vi "Adressen.vi"(8 "error in (no error)":errorcluster caption="Fehler (Eingang, kein Fehler)", 11 "Schneider Steuerung PNS Eingang":refnum<class "Schneider Steuerung PNS.lvclass">) -> (0 "error out":errorcluster caption="Fehler (Ausgang)", 2 "Adressen out":T1, 3 "Schneider Steuerung PNS Ausgang":refnum<class "Schneider Steuerung PNS.lvclass">)   [LabVIEW 2020, in "Schneider Steuerung PNS.lvclass"]
uses:
  Schneider Steuerung PNS.lvclass
  Adresse.ctl
  Steuerung PNS.lvclass
panel:
  in  "Adressen IP":i32[](array[numeric])=[4000, 4001, 4002, 4003, 4090]
  in  "Alarm":i32[](array[numeric])=[300, 200, 301, 201, 302, 202, 303, 203, 304, 204, 305, 205, 306, 206, 307, 207]
  in  "Heizkreiserkennung":i32[](array[numeric])=[520, 521, 522, 523, 524, 525, 526, 527]
  in  "Allgemein":i32[](array[numeric])=[504, 506, 503, 502, 501, 500, 870, 4976, 505, 4977, 4978, 4979, 4980, 5000, 5002]
  in  "Loop 8":i32[](array[numeric])=[407, 7, 207, 307, 457, 107]
  in  "Loop 7":i32[](array[numeric])=[406, 6, 206, 306, 456, 106]
  in  "Loop 6":i32[](array[numeric])=[405, 5, 205, 305, 455, 105]
  in  "Loop 5":i32[](array[numeric])=[404, 4, 204, 304, 454, 104]
  in  "Loop 4":i32[](array[numeric])=[403, 3, 203, 303, 453, 103]
  in  "Loop 3":i32[](array[numeric])=[402, 2, 202, 302, 452, 102]
  in  "Loop 2":i32[](array[numeric])=[401, 1, 201, 301, 451, 101]
  in  "Loop 1":i32[](array[numeric])=[400, 8, 200, 300, 450, 100]
  # "Istwert\n\nSollwert\n\nAlarm MIN\n\nAlarm MAX\n\nRegler sperren\n\nAnalog Ausgang"
  # "AWC ist\n\nAusgang Prop.\n\nAuswahl NW/M/BP\n\nAWC Netzwerk\n\nAWC Manuell\n\nAWC Bitparallel\n\nDruckluft störung\n\nGeräte Erkennung\n\nGeräte Type\n\nSeriennummer\n\nIB-Jahr\n\nSoftWare Version\n\nLP Kennung\n\nVentile Schalten\n\nVentilstellung Anzeige"
  # "Benennung Heizkreis 1\n\nBenennung Heizkreis 2\n\nBenennung Heizkreis 3\n\nBenennung Heizkreis 4\n\nBenennung Heizkreis 5\n\nBenennung Heizkreis 6\n\nBenennung Heizkreis 7\n\nBenennung Heizkreis 8"
  # "Alarm Filter max\n\nAlarm Filter min\n\nAlarm Ventilplatte max\n\nAlarm Ventilplatte min\n\nAlarm HL1 max\n\nAlarm HL1 min\n\nAlarm HL2 max\n\nAlarm HL2 min\n\nAlarm HL3 max\n\nAlarm HL3 min\n\nAlarm HL4 max\n\nAlarm HL4 min\n\nAlarm HL5 max\n\nAlarm HL5 min\n\nAlarm HL6 max\n\nAlarm HL6 min"
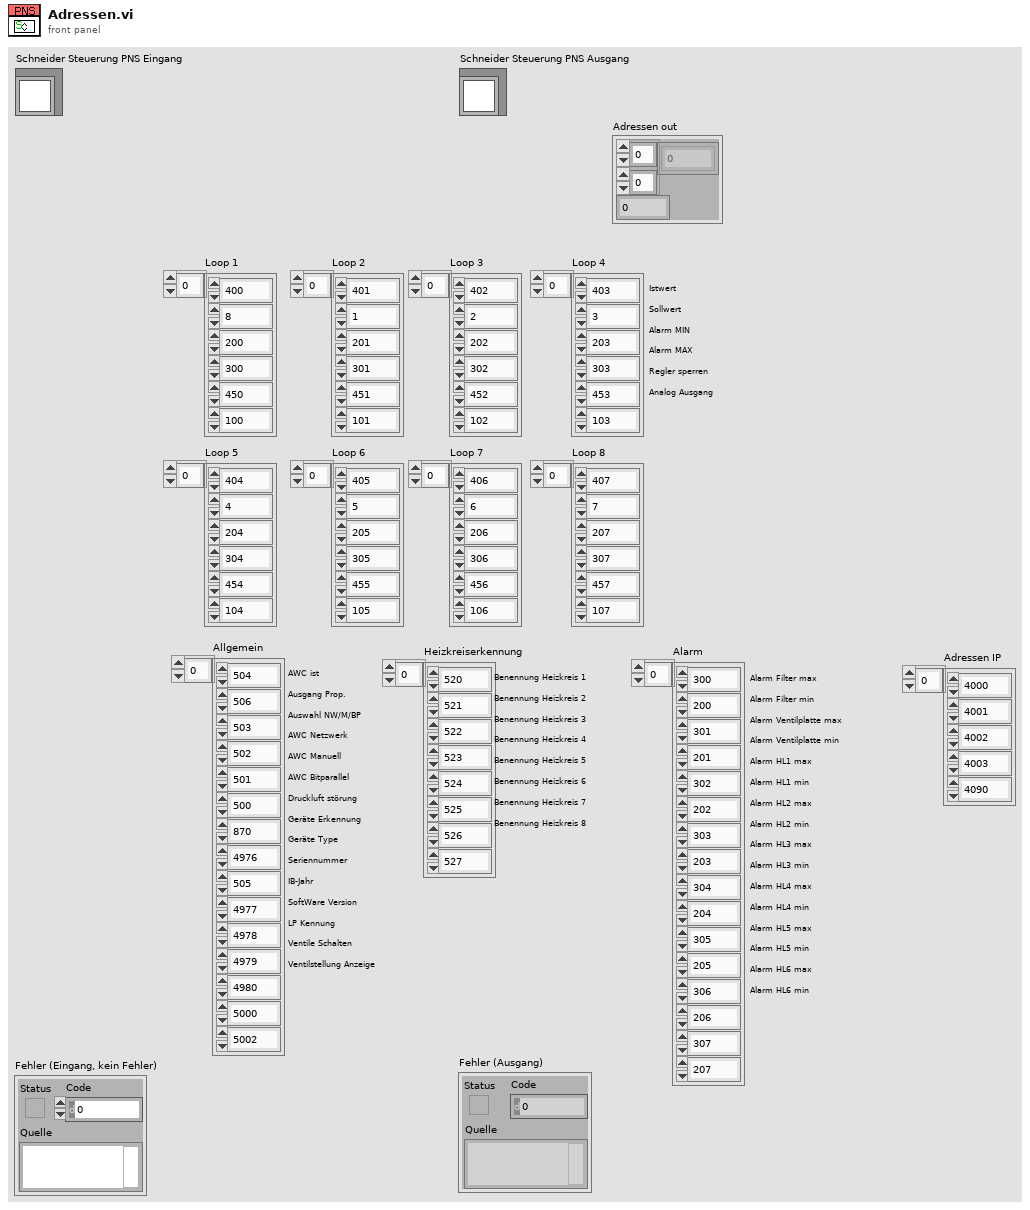
[diagram p1: front panel]
types:
  T1 = typedef "Steuerung PNS.lvclass/Adresse.ctl" = cluster{i32[][], i32}
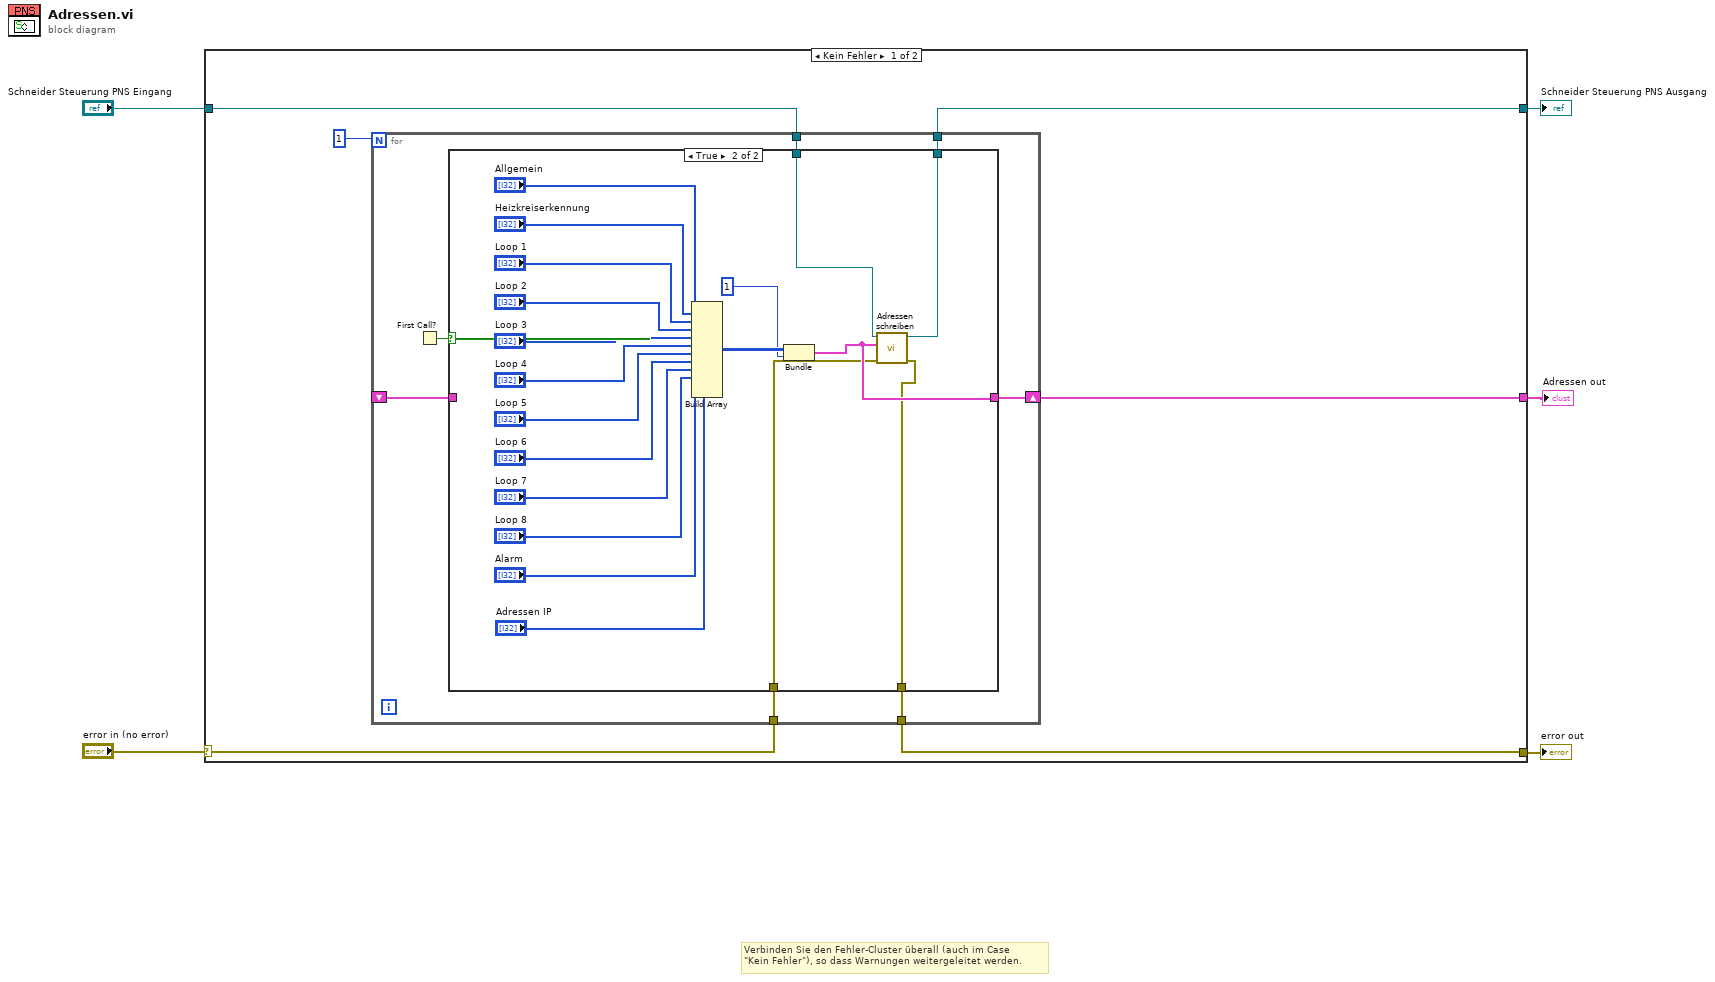
[diagram p0: block diagram]
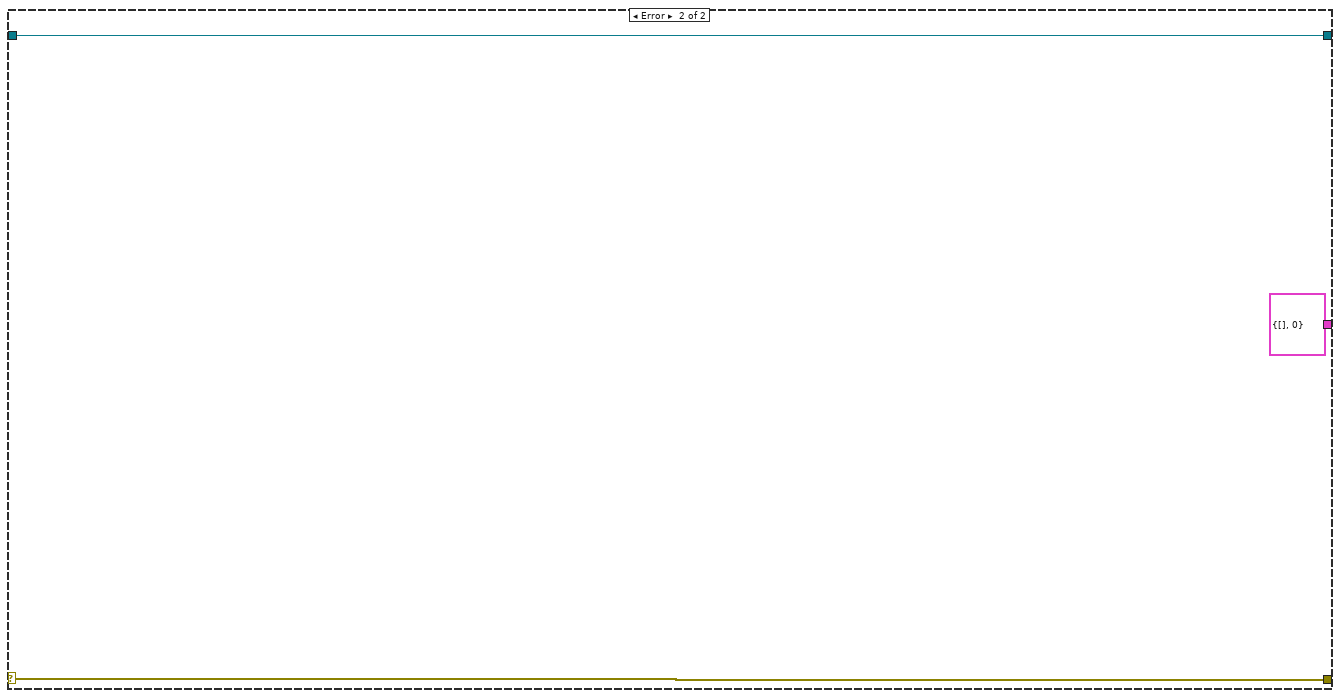
[diagram p3: hidden frame]
diagram:
  # "Verbinden Sie den Fehler-Cluster überall (auch im Case\n\"Kein Fehler\"), so dass Warnungen weitergeleitet werden."
  n1 = case shown="Kein Fehler" "error in (no error)" {
    selector: "error in (no error)" -> [w7 w43]
    tunnel: [w6 w43] -> w4
    tunnel: [w8 w42] -> w2
    tunnel: "Schneider Steuerung PNS Eingang" -> [w9 w42]
    tunnel: [w10 cluster{i32[][], i32} {[], 0} ("Adressen out")] -> w1
    frame No Error {
      n2 = for {
        N: 1 -> [_]
        shift-right: [w17] -> w10
        shift-left: _ -> [w16]
        tunnel: w9 -> [w15]
        tunnel: [w14] -> w8
        tunnel: [w13] -> w6
        tunnel: w7 -> [w12]
        n3 = First Call?() -> (First Call?: T/F=w18:bool)
        n4 = case shown="True" w18 {
          tunnel: [w21 w27] -> w17
          tunnel: w16 -> [w21 _]
          tunnel: w15 -> [w20 w26]
          tunnel: [w20 w25] -> w14
          tunnel: [w19 w24] -> w13
          tunnel: w12 -> [w19 w23]
          frame False {
          }
          frame True {
            n5 = Build Array("Allgemein", "Heizkreiserkennung", "Loop 1", "Loop 2", "Loop 3", "Loop 4", "Loop 5", "Loop 6", "Loop 7", "Loop 8", "Alarm", "Adressen IP") -> (w29:i32[][])
            n6 = Bundle(w29, 1) -> (w27:cluster{i32[][], i32})  [unwired: 1 in]
            n7 = call-dynamic "Adressen schreiben.vi"("error in (no error)"=w23, "Adressen"=w27, "Steuerung PNS (Eingang)"=w26) -> ("error out"=w24:errorcluster, "Steuerung PNS (Ausgang)"=w25:refnum<class "Schneider Steuerung PNS.lvclass">)  [unwired: 7 in]
          }
        }
      }
    }
    frame Error {
    }
  }
  "error out" <- w4
  "Schneider Steuerung PNS Ausgang" <- w2
  "Adressen out" <- w1
